vi "GetBounds.vi"(0 "XRef":T5, 1 "State In":T4) -> (14 "Bounds":T2, 15 "Fatal Error Out":T1)   [LabVIEW 2015, in "Set Object Parameters.xnode"]
uses:
  Set Object Parameters.xnode
  <vilib>/XNodeSupport/XNodeXNodeRef.ctl
  State.ctl
  <vilib>/XNodeSupport/XNodeBounds.ctl
  <vilib>/XNodeSupport/XNodeInt.ctl
  <vilib>/XNodeSupport/XNodeErrorCluster.ctl
  dimensions.vi
  <vilib>/XNodeSupport/NI_XNodeSupport.lvlib
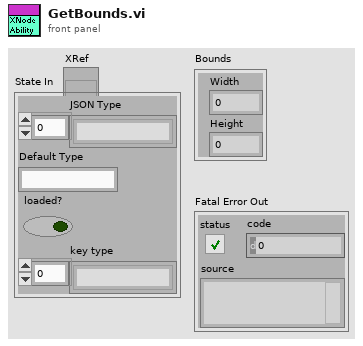
[diagram p1: front panel]
types:
  T1 = typedef "NI_XNodeSupport.lvlib/XNodeErrorCluster.ctl" = errorcluster
  T2 = typedef "NI_XNodeSupport.lvlib/XNodeBounds.ctl" = cluster{"Width":T3, "Height":T3}
  T3 = typedef "NI_XNodeSupport.lvlib/XNodeInt.ctl" = i32
  T4 = typedef "Set Object Parameters.xnode/State.ctl" = cluster{"JSON Type":string[], "Default Type":string, "loaded?":bool, "key type":string[]}
  T5 = typedef "NI_XNodeSupport.lvlib/XNodeXNodeRef.ctl" = refnum<vi>
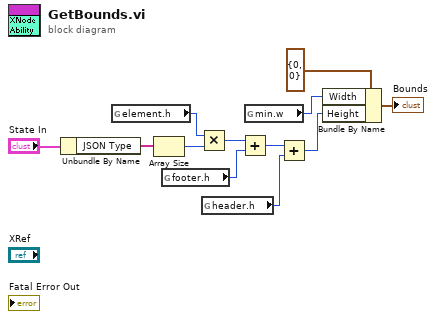
[diagram p0: block diagram]
diagram:
  n1 = Unbundle By Name("State In") -> ("JSON Type"=w2:string[])
  n2 = global read "dimensions.vi" "element.h"() -> (w8:i16)
  n3 = Array Size(array=w2) -> (size(s)=w1:i32)
  n4 = global read "dimensions.vi" "footer.h"() -> (w6:i16)
  n5 = Multiply(x=w8, y=w1) -> (x*y=w7:i32)
  n6 = global read "dimensions.vi" "header.h"() -> (w4:i16)
  n7 = Add(x=w7, y=w6) -> (x+y=w5:i32)
  n8 = global read "dimensions.vi" "min.w"() -> (w10:i32)
  n9 = Add(x=w5, y=w4) -> (x+y=w3:i32)
  n10 = Bundle By Name(cluster=T2 {"Width"=0, "Height"=0} ("Bounds"), "Width"=w10, "Height"=w3) -> (→"Bounds":T2)
